vi "Sample--Sync_MasterSlaveRefClk_USB.vi"() -> ()   [LabVIEW 2013]
doc: "This example demonstrates synchronizing two digitizers."
uses:
  <userlib>/ArtScope/Trigger/ArtScope_ConfigureTriggerDigital.vi
  <userlib>/ArtScope/Fetch/ArtScope_FetchBinary16.vi
  <userlib>/ArtScope/_SubVI/ArtScope_ArrayByChannel_U16.vi
panel:
  out "error out":errorcluster
  in  "reference position2":dbl
  in  "reference position":dbl
  in  "range2(Vpp)":i32(ring) items=["20V", "10V", "2V", "40V", "16V", "8V", "4V", "1.6V", "800m", "400m", "160m", "80m", "40m"]
  in  "range(Vpp)":i32(ring) items=["20V", "10V", "2V", "40V", "16V", "8V", "4V", "1.6V", "800m", "400m", "160m", "80m", "40m"]
  in  "Slave":string="Dev2"
  in  "Master":string="Dev1"
  in  "Stop":bool
  out "Data2":u16[][](graph)
  in  "Timeout(s) 2":dbl=1.0
  in  "MinSampleRate 2":dbl=8000000.0
  in  "MinRecordLength2":i32=6000
  out "Data":u16[][](graph)
  in  "Timeout(s)":dbl=1.0
  in  "MinRecordLength":i32=6000
  in  "MinSampleRate":dbl=8000000.0
  # "Vertical"
  # "Horizontal"
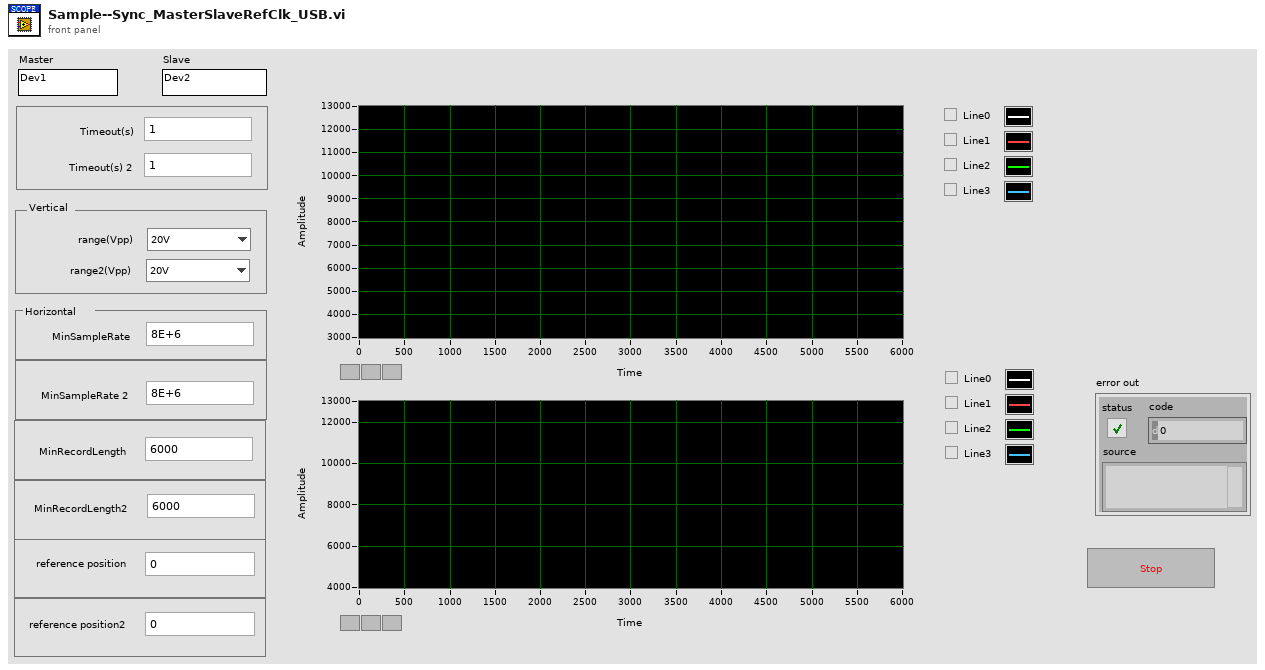
[diagram p1: front panel]
types:
  T1 = cluster{"fLSB":cluster{dbl, dbl, dbl, dbl, dbl, dbl, dbl, dbl}, "RangeValue":cluster{dbl, dbl, dbl, dbl, dbl, dbl, dbl, dbl}, "wMaxLSB":u32, "TriggerMode":i32, "sampLengthPerChan":u32, "pAvailSampsPoints":u32, "channelCount":i32}
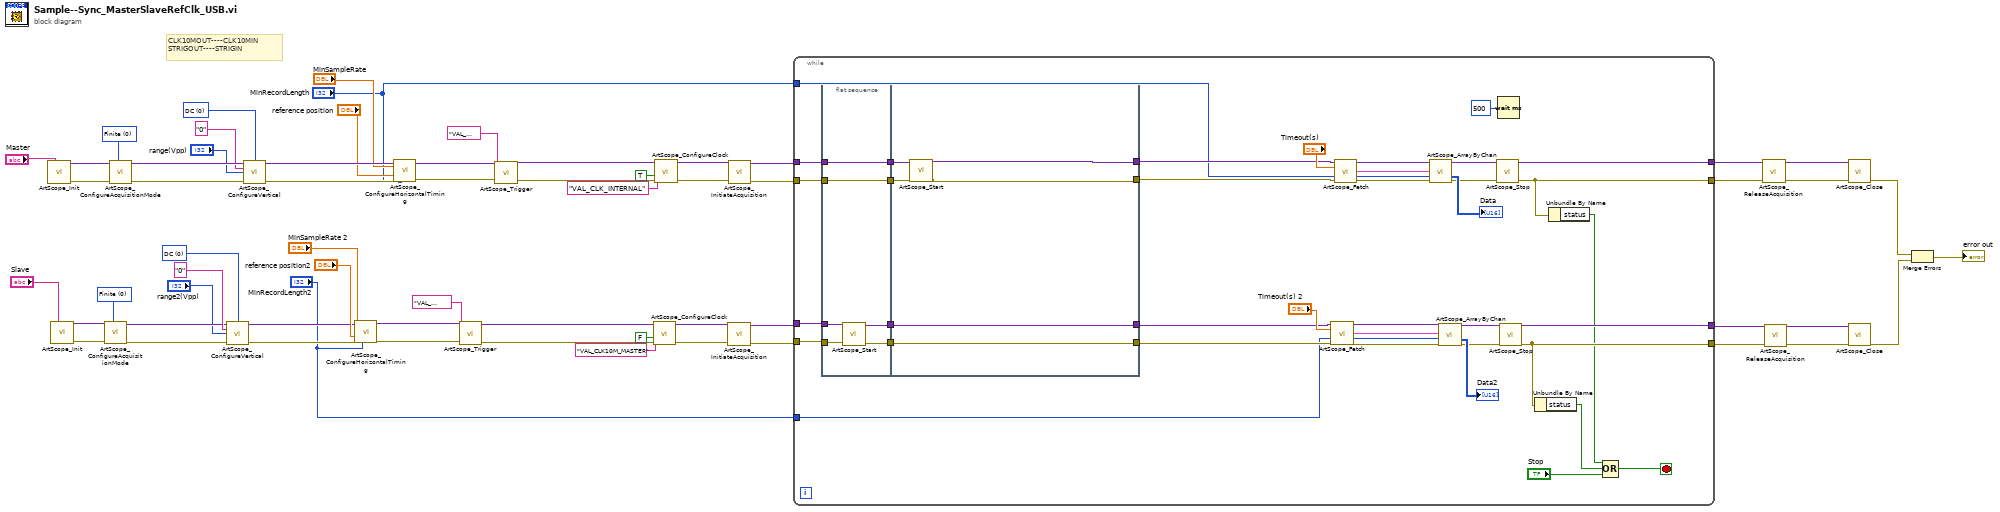
[diagram p0: block diagram]
diagram:
  w44 = 0 items=["DC", "AC"] ("Coupling")
  w50 = 0 items=["Finite", "Continuous"] ("AcuqMode")
  w59 = 0 items=["DC", "AC"] ("Coupling")
  w54 = 0 items=["Finite", "Continuous"] ("AcuqMode")
  # "CLK10MOUT----CLK10MIN\nSTRIGOUT----STRIGIN"
  n1 = call <userlib>:"ArtScope_Init.vi"("task name"="Master") -> ("task handle"=w41:variant, "error out"=w40:errorcluster)  [unwired: 13 in]
  n2 = call <userlib>:"ArtScope_Init.vi"("task name"="Slave") -> ("task handle"=w38:variant, "error out"=w37:errorcluster)  [unwired: 13 in]
  n3 = call <userlib>:"ArtScope_ConfigureAcquisitionMode.vi"("task handle"=w38, "acquisition mode"=w50, "error in (no error)"=w37) -> ("task handle"=w43:variant, "error out"=w42:errorcluster)  [unwired: 11 in]
  n4 = call <userlib>:"ArtScope_ConfigureAcquisitionMode.vi"("task handle"=w41, "acquisition mode"=w54, "error in (no error)"=w40) -> ("task handle"=w53:variant, "error out"=w55:errorcluster)  [unwired: 11 in]
  n5 = call <userlib>:"ArtScope_ConfigureVertical.vi"("task handle"=w43, "coupling"=w44, "channels"="0" ("Channel Name"), "range(Vpp)"="range2(Vpp)", "error in (no error)"=w42) -> ("task handle"=w45:variant, "error out"=w46:errorcluster)  [unwired: 9 in]
  n6 = call <userlib>:"ArtScope_ConfigureVertical.vi"("task handle"=w53, "coupling"=w59, "channels"="0" ("Channel Name"), "range(Vpp)"="range(Vpp)", "error in (no error)"=w55) -> ("task handle"=w58:variant, "error out"=w57:errorcluster)  [unwired: 9 in]
  n7 = call <userlib>:"ArtScope_ConfigureHorizontalTiming.vi"("task handle"=w45, "min sample rate"="MinSampleRate 2", "reference position"="reference position2", "error in (no error)"=w46, "min record length"="MinRecordLength2") -> ("task handle"=w14:variant, "error out"=w13:errorcluster)  [unwired: 9 in]
  n8 = call <userlib>:"ArtScope_ConfigureHorizontalTiming.vi"("task handle"=w58, "min sample rate"="MinSampleRate", "reference position"="reference position", "error in (no error)"=w57, "min record length"="MinRecordLength") -> ("task handle"=w11:variant, "error out"=w10:errorcluster)  [unwired: 9 in]
  n9 = call-poly <userlib>:"ArtScope_Trigger.vi"("task handle"=w14, "trigger source"="VAL_TRIGGER_SYNCTRIGGER", "error in"=w13) -> ("task handle"=w5:variant, "error out"=w4:errorcluster)  [unwired: 11 in]
  n10 = call-poly <userlib>:"ArtScope_Trigger.vi"("task handle"=w11, "trigger source"="VAL_TRIGGER_DTR", "error in"=w10) -> ("task handle"=w6:variant, "error out"=w7:errorcluster)  [unwired: 11 in]
  n11 = call <userlib>:"ArtScope_ConfigureClock.vi"("task handle"=w5, "input clock source"="VAL_CLK10M_MASTER", "master enable"=FALSE, "error in (no error)"=w4) -> ("task handle"=w35:variant, "error out"=w33:errorcluster)  [unwired: 10 in]
  n12 = call <userlib>:"ArtScope_ConfigureClock.vi"("task handle"=w6, "input clock source"="VAL_CLK_INTERNAL", "master enable"=TRUE ("ClkOutEnable"), "error in (no error)"=w7) -> ("task handle"=w29:variant, "error out"=w31:errorcluster)  [unwired: 10 in]
  n13 = call <userlib>:"ArtScope_InitiateAcquisition.vi"("task handle"=w35, "error in (no error)"=w33) -> ("task handle"=w34:variant, "error out"=w32:errorcluster)  [unwired: 12 in]
  n14 = call <userlib>:"ArtScope_InitiateAcquisition.vi"("task handle"=w29, "error in (no error)"=w31) -> ("task handle"=w28:variant, "error out"=w30:errorcluster)  [unwired: 12 in]
  n15 = while {
    tunnel: [w98] -> w27
    tunnel: [w85] -> w25
    tunnel: [w87] -> w23
    tunnel: [w97] -> w20
    tunnel: w34 -> [w96]
    tunnel: w32 -> [w95]
    tunnel: w28 -> [w91]
    tunnel: w30 -> [w90]
    tunnel: "MinRecordLength" -> [w77]
    tunnel: "MinRecordLength2" -> [w76]
    stop <- w82 stop-if-true
    n16 = flat-sequence {
      tunnel: w96 -> [w106]
      tunnel: w95 -> [w105]
      tunnel: [w101] -> w100
      tunnel: [w104] -> w99
      tunnel: [w103] -> w92
      tunnel: w91 -> [w103]
      tunnel: w90 -> [w102]
      tunnel: [w102] -> w89
      tunnel: w100 -> [w112]
      tunnel: w99 -> [w111]
      tunnel: w92 -> [w110]
      tunnel: w89 -> [w109]
      tunnel: [w107] -> w80
      tunnel: [w108] -> w81
      tunnel: [w112] -> w79
      tunnel: [w111] -> w78
      frame #0 {
        n17 = call <userlib>:"ArtScope_Start.vi"("task handle"=w106, "error in (no error)"=w105) -> ("task handle"=w101:variant, "error out"=w104:errorcluster)  [unwired: 12 in]
      }
      frame #1 {
        n18 = call <userlib>:"ArtScope_Start.vi"("task handle"=w110, "error in (no error)"=w109) -> ("task handle"=w108:variant, "error out"=w107:errorcluster)  [unwired: 12 in]
      }
    }
    n19 = call-poly <userlib>:"ArtScope_Fetch.vi"("task handle"=w79, "timeout"="Timeout(s) 2", "num samples"=w76, "error in (no error)"=w78) -> ("task handle"=w67:variant, "wfm info"=w63:T1, "data"=w62:u16[], "error out"=w64:errorcluster)  [unwired: 8 in]
    n20 = call-poly <userlib>:"ArtScope_Fetch.vi"("task handle"=w81, "timeout"="Timeout(s)", "num samples"=w77, "error in (no error)"=w80) -> ("task handle"=w73:variant, "wfm info"=w69:T1, "data"=w68:u16[], "error out"=w72:errorcluster)  [unwired: 8 in]
    n21 = call-poly <userlib>:"ArtScope_ArrayByChan.vi"("task handle"=w73, "wfm info"=w69, "1D data"=w68, "error in (no error)"=w72) -> ("task handle"=w70:variant, "2D data"=→"Data":u16[][], "error out"=w71:errorcluster)  [unwired: 9 in]
    n22 = call-poly <userlib>:"ArtScope_ArrayByChan.vi"("task handle"=w67, "wfm info"=w63, "1D data"=w62, "error in (no error)"=w64) -> ("task handle"=w66:variant, "2D data"=→"Data2":u16[][], "error out"=w65:errorcluster)  [unwired: 9 in]
    n23 = call <userlib>:"ArtScope_Stop.vi"("task handle"=w70, "error in"=w71) -> ("task handle"=w98:variant, "error out"=w85:errorcluster)  [unwired: 12 in]
    n24 = Wait (ms)(milliseconds to wait=u32 500 ("等待时间（毫秒）")) -> ()  [unwired: 1 out]
    n25 = call <userlib>:"ArtScope_Stop.vi"("task handle"=w66, "error in"=w65) -> ("task handle"=w97:variant, "error out"=w87:errorcluster)  [unwired: 12 in]
    n26 = Unbundle By Name(w87) -> ("status"=w86:bool)
    n27 = Unbundle By Name(w85) -> ("status"=w84:bool)
    n28 = Compound Arithmetic op=OR(w84, w86, "Stop") -> (w82:bool)
  }
  n29 = call <userlib>:"ArtScope_ReleaseAcquisition.vi"("task handle"=w27, "error in (no error)"=w25) -> ("task handle"=w26:variant, "error out"=w24:errorcluster)  [unwired: 12 in]
  n30 = call <userlib>:"ArtScope_ReleaseAcquisition.vi"("task handle"=w20, "error in (no error)"=w23) -> ("task handle"=w21:variant, "error out"=w22:errorcluster)  [unwired: 12 in]
  n31 = call <userlib>:"ArtScope_Close.vi"("task handle"=w26, "error in (no error)"=w24) -> ("error out"=w61:errorcluster)  [unwired: 13 in]
  n32 = call <userlib>:"ArtScope_Close.vi"("task handle"=w21, "error in (no error)"=w22) -> ("error out"=w60:errorcluster)  [unwired: 13 in]
  n33 = Merge Errors(w61, w60) -> (→"error out":errorcluster)
